vi "Set_Channel_Coeff_client.vi"() -> ()   [LabVIEW 2017]
doc: "This is an example of using features of the VI Server as a client. It shows how you might browse from one or more applications that may be exporting data from one or more data stations. \n\nThe example shows how to query a server for its list of exported VIs, how to get references to the VIs, and how call them with the Call By Reference function."
uses:
  Anemometry/Anemometry Sub Vis/Globals/Preference_global.vi
panel:
  in  "Set Array":T1(array[cluster]) {"Set value of D to" format="%.2f"; "Set value of C to" format="%.2f"; "Set value of B to" format="%.2f"; "Set value of A to" format="%.2f"}
  in  "server type":refnum<vi>
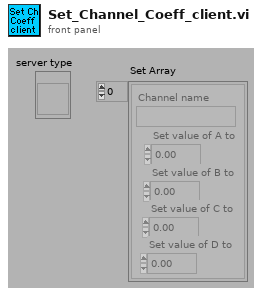
[diagram p1: front panel]
types:
  T1 = cluster{"Channel name":string, "Set value of A to":dbl, "Set value of B to":dbl, "Set value of C to":dbl, "Set value of D to":dbl}[]
  T2 = typedef "Server_Comms.ctl" = enum16{"Server Link Healthy", "Do Not Link To Server"}
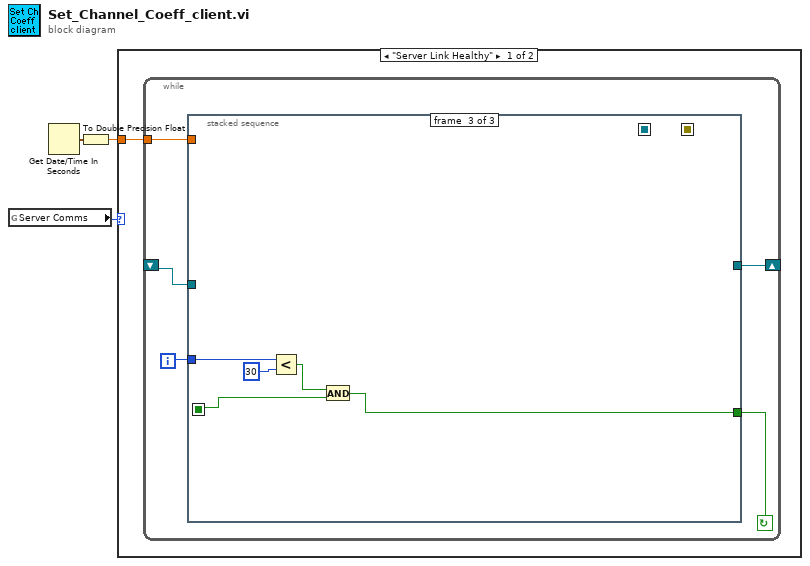
[diagram p0: block diagram]
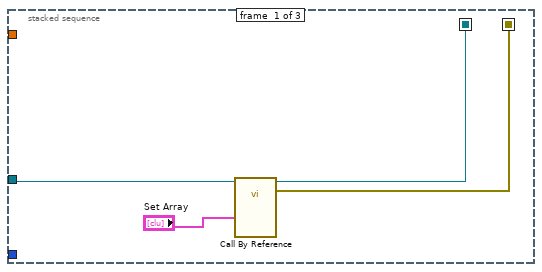
[diagram p2: hidden frame]
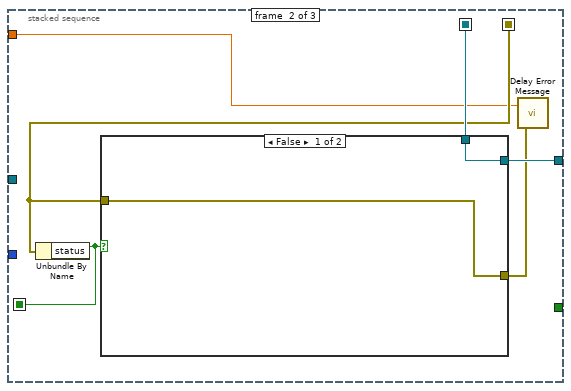
[diagram p3: hidden frame]
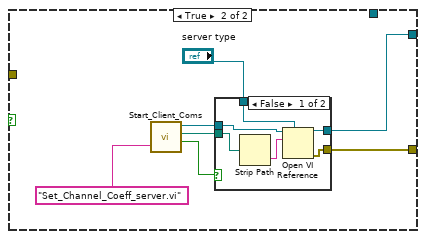
[diagram p4: hidden frame]
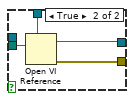
[diagram p5: hidden frame]
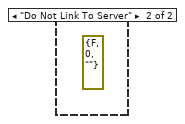
[diagram p6: hidden frame]
diagram:
  n1 = global read "Preference_global.vi" "Server Comms"() -> (w3:T2)
  n2 = Get Date/Time In Seconds() -> (seconds since 1Jan1904=w2:timestamp)
  n3 = To Double Precision Float(number=w2) -> (double precision float=w1:dbl)
  n4 = case shown="\"Server Link Healthy\"" w3 {
    tunnel: w1 -> [w4 _]
    frame "Server Link Healthy" {
      n5 = while {
        shift-left: _ -> [w9]
        shift-right: [w8] -> _
        tunnel: w4 -> [w5]
        i -> [w7]
        stop <- w6 continue-if-true
        n6 = stacked-sequence {
          seq-local: [w11 _ _] -> [_ w18 _]
          seq-local: [w12 _ _] -> [_ w16 _]
          seq-local: [_ w17 _] -> [_ _ w40]
          tunnel: w9 -> [w10 _ _]
          tunnel: [_ w19 _] -> w8
          tunnel: w7 -> [_ _ w41]
          tunnel: [_ _ w39] -> w6
          tunnel: w5 -> [_ w14 _]
          frame #0 {
            n7 = call-by-ref "?"(reference=w10, "Set Array"="Set Array") -> (reference out=w11:refnum<vi>, error out=w12:errorcluster)  [unwired: 1 in]
          }
          frame #1 {
            n8 = Unbundle By Name(w16) -> ("status"=w17:bool)
            n9 = case shown="False" w17 {
              tunnel: [w21 w24] -> w19
              tunnel: w18 -> [w21 _]
              tunnel: [w20 w22] -> w15
              tunnel: w16 -> [w20 _]
              frame False {
              }
              frame True {
                n10 = call "Start_Client_Coms.vi"("VI name to run on server"="Set_Channel_Coeff_server.vi") -> ("LabVIEW application reference"=w26:refnum<vi>, "Checked VI name"=w27:path, "Local Call"=w25:bool)  [unwired: 1 in, 1 out]
                n11 = case shown="False" w25 {
                  tunnel: [w33 w38] -> w24
                  tunnel: "server type" -> [w31 w37]
                  tunnel: w27 -> [w30 w36]
                  tunnel: w26 -> [w29 _]
                  tunnel: [w32 w35] -> w22
                  frame False {
                    n12 = Strip Path(path=w30) -> (name=w34:string)  [unwired: 1 out]
                    n13 = Open VI Reference(type specifier VI Refnum (for type only)=w31, application reference (local)=w29, vi path=w34) -> (vi reference=w33:refnum<vi>, error out=w32:errorcluster)  [unwired: 1 in, 2 out]
                  }
                  frame True {
                    n14 = Open VI Reference(type specifier VI Refnum (for type only)=w37, vi path=w36) -> (vi reference=w38:refnum<vi>, error out=w35:errorcluster)  [unwired: 1 in, 3 out]
                  }
                }
              }
            }
            n15 = call "Delay Error Message.vi"("error in (no error)"=w15, "Seconds since 1904"=w14) -> ()  [unwired: 2 in]
          }
          frame #2 {
            n16 = Less?(x=w41, y=30) -> (x < y?=w43:bool)
            n17 = And(x=w43, y=w40) -> (x .and. y?=w39:bool)
          }
        }
      }
    }
    frame "Do Not Link To Server" {
      (unwired) errorcluster {"status"=FALSE, "code"=0, "source"=""}
    }
  }
